vi "Icon.vi"(11 "ZIP Item in":refnum<class "ZIP Item.lvclass">) -> (2 "Icon":T1 caption="Icon (16x16 px)")   [LabVIEW 2019, in "ZIP.lvlib" / "ZIP Item.lvclass"]
uses:
  ZIP Item.lvclass
  libs/Solution.lvlibp/1abvi3w/vi.lib/picture/picture.llb/imagedata.ctl
  libs/Solution.lvlibp
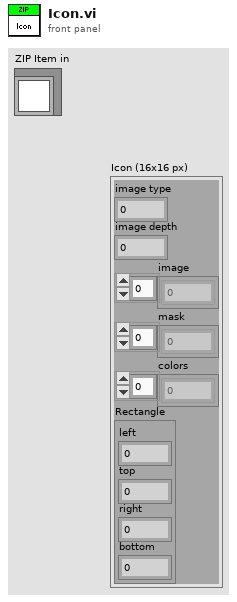
[diagram p1: front panel]
types:
  T1 = typedef "Solution.lvlibp/imagedata.ctl" = cluster{"image type":i32, "image depth":i32, "image":u8[], "mask":u8[], "colors":u32[], "Rectangle":cluster{"left":i16, "top":i16, "right":i16, "bottom":i16}}
  T2 = cluster{"image type":i32, "image depth":i32, "image":u8[], "mask":u8[], "colors":u32[], "Rectangle":cluster{"left":i16, "top":i16, "right":i16, "bottom":i16}}
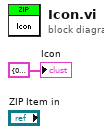
[diagram p0: block diagram]
diagram:
  "Icon" <- T2 {"image type"=0, "image depth"=24, "image"=[255, 255, 255, 255, 255, 255, 255, 255, 255, 255, 255, 255, 255, 255, 255, 255, 255, 255, 255, 255, 255, 41, 100, 169, 55, 115, 185, 107, 160, 213, 51, 110, 180, 255, 255, 255, 255, 255, 255, 255, 255, 255, 255, 255, 255, 255, 255, 255, 255, 255, 255, 255, 255, 255, 255, 255, 255, 255, 255, 255, 255, 255, 255, 255, 255, 255, 41, 100, 169, 55, 115, 185, 107, 160, 213, 51, 110, 180, 255, 255, 255, 255, 255, 255, 255, 255, 255, 255, 255, 255, 255, 255, 255, 166, 166, 166, 171, 171, 114, 171, 171, 114, 167, 166, 130, 85, 96, 102, 171, 192, 204, 171, 192, 204, 171, 192, 204, 171, 192, 204, 171, 192, 204, 171, 192, 204, 122, 162, 203, 102, 136, 177, 255, 255, 255, 214, 190, 45, 140, 140, 140, 223, 210, 106, 221, 209, 83, 221, 209, 83, 98, 104, 83, 50, 75, 98, 50, 75, 98, 50, 75, 98, 50, 75, 98, 50, 75, 98, 48, 89, 133, 62, 104, 151, 136, 182, 219, 97, 132, 174, 214, 190, 45, 214, 218, 214, 243, 239, 205, 243, 239, 205, 240, 231, 177, 240, 228, 162, 235, 223, 142, 233, 220, 126, 233, 217, 112, 234, 217, 106, 212, 196, 100, 55, 61, 53, 127, 151, 174, 136, 182, 219, 30, 86, 149, 214, 190, 45, 218, 223, 204, 251, 232, 90, 248, 229, 85, 242, 217, 63, 238, 211, 51, 235, 206, 42, 235, 206, 42, 233, 203, 37, 233, 203, 37, 229, 201, 37, 79, 76, 37, 127, 151, 174, 136, 182, 219, 30, 86, 149, 214, 190, 45, 217, 220, 187, 244, 225, 84, 243, 218, 65, 235, 206, 42, 233, 203, 37, 233, 203, 37, 232, 201, 30, 232, 201, 30, 232, 201, 30, 231, 200, 30, 86, 80, 34, 127, 151, 174, 136, 182, 219, 30, 86, 149, 214, 190, 45, 218, 214, 147, 240, 214, 55, 235, 206, 42, 232, 201, 30, 232, 201, 30, 232, 201, 30, 232, 201, 30, 232, 201, 30, 232, 201, 30, 231, 200, 30, 79, 76, 37, 127, 151, 174, 136, 182, 219, 30, 86, 149, 214, 190, 45, 220, 208, 102, 233, 203, 37, 233, 203, 37, 223, 196, 39, 223, 196, 39, 223, 196, 39, 223, 196, 39, 223, 196, 39, 223, 196, 39, 223, 196, 39, 68, 69, 45, 127, 151, 174, 136, 182, 219, 30, 86, 149, 214, 190, 45, 223, 204, 68, 232, 201, 30, 233, 203, 37, 238, 211, 51, 242, 217, 63, 246, 225, 77, 248, 229, 85, 251, 232, 90, 251, 232, 90, 219, 207, 85, 50, 58, 56, 127, 151, 174, 136, 182, 219, 30, 86, 149, 214, 190, 45, 223, 204, 68, 233, 203, 37, 235, 206, 42, 242, 220, 73, 244, 225, 84, 247, 229, 92, 248, 231, 97, 246, 231, 98, 246, 231, 98, 217, 208, 88, 50, 58, 56, 127, 151, 174, 136, 182, 219, 30, 86, 149, 214, 190, 45, 153, 153, 153, 153, 153, 153, 153, 153, 153, 50, 86, 103, 35, 80, 95, 33, 66, 76, 33, 54, 64, 33, 54, 64, 33, 54, 64, 33, 54, 64, 16, 27, 32, 113, 139, 165, 136, 182, 219, 30, 86, 149, 255, 255, 255, 255, 255, 255, 255, 255, 255, 255, 255, 255, 97, 132, 174, 171, 192, 204, 171, 192, 204, 171, 192, 204, 171, 192, 204, 171, 192, 204, 171, 192, 204, 171, 192, 204, 104, 142, 179, 94, 146, 198, 89, 120, 158, 255, 255, 255, 255, 255, 255, 255, 255, 255, 255, 255, 255, 255, 255, 255, 56, 111, 173, 42, 96, 157, 35, 61, 88, 48, 89, 133, 61, 116, 178, 93, 143, 191, 42, 96, 157, 42, 96, 157, 94, 126, 162, 255, 255, 255, 255, 255, 255, 255, 255, 255, 255, 255, 255, 255, 255, 255, 255, 255, 255, 255, 255, 255, 255, 255, 255, 81, 125, 176, 55, 115, 185, 85, 140, 199, 76, 130, 188, 255, 255, 255, 255, 255, 255, 255, 255, 255, 255, 255, 255, 255, 255, 255, 255, 255, 255, 255, 255, 255, 255, 255, 255, 255, 255, 255, 255, 255, 255, 255, 255, 255, 81, 125, 176, 55, 115, 185, 85, 140, 199, 76, 130, 188, 255, 255, 255, 255, 255, 255, 255, 255, 255, 255, 255, 255], "mask"=[], "colors"=[], "Rectangle"={"left"=0, "top"=0, "right"=15, "bottom"=16}}
